vi "Write Log Path.vi"(8 "error in (no error)":errorcluster, 10 "Log Path":path, 11 "Actor_log in":refnum<class "Actor_log.lvclass">) -> (0 "error out":errorcluster, 3 "Actor_log out":refnum<class "Actor_log.lvclass">)   [LabVIEW 2020, in "Actor_log.lvlib" / "Actor_log.lvclass"]
uses:
  Actor_log.lvclass
  Actor_log.lvclass/Actor_log.ctl
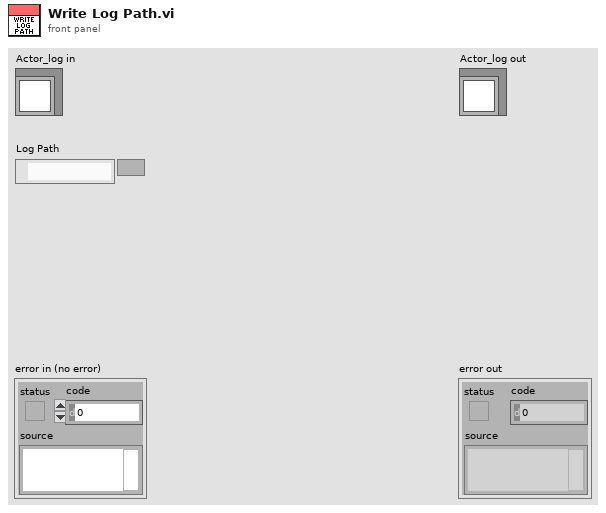
[diagram p1: front panel]
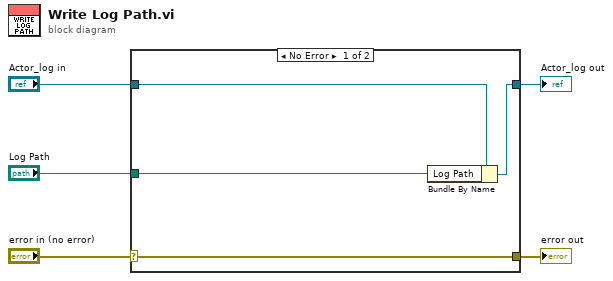
[diagram p0: block diagram]
diagram:
  n1 = case shown="No Error" "error in (no error)" {
    selector: "error in (no error)" -> [w9 w10]
    tunnel: [w9 w10] -> w4
    tunnel: [w7 w11] -> w2
    tunnel: "Actor_log in" -> [w8 w11]
    tunnel: "Log Path" -> [w6 _]
    frame No Error {
      n2 = Bundle By Name(cluster=w8, "Log Path"=w6) -> (w7:refnum<class "Actor_log.lvclass">)
    }
    frame Error {
    }
  }
  "error out" <- w4
  "Actor_log out" <- w2
